vi "Track.vi"() -> ()   [LabVIEW 2014]
uses:
  <vilib>/Instr/_visa.llb/VISA Flush IO Buffer Mask.ctl
  <vilib>/Instr/_visa.llb/VISA Configure Serial Port (Instr).vi
panel:
  out "Direction":bool
  out "Whale?":bool
  out "read buffer":string
  out "return count":u32
  in  "stop":bool
  in  "VISA resource name":refnum<visa-resource-name>="COM3"
  in  "Base":dbl[][](array[numeric])
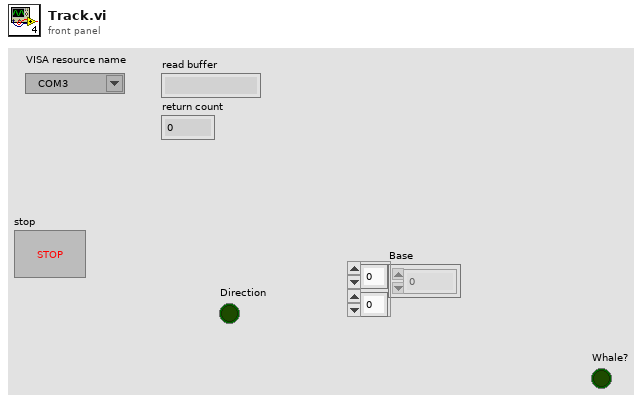
[diagram p1: front panel]
types:
  T1 = typedef "VISA Flush IO Buffer Mask.ctl" = u16
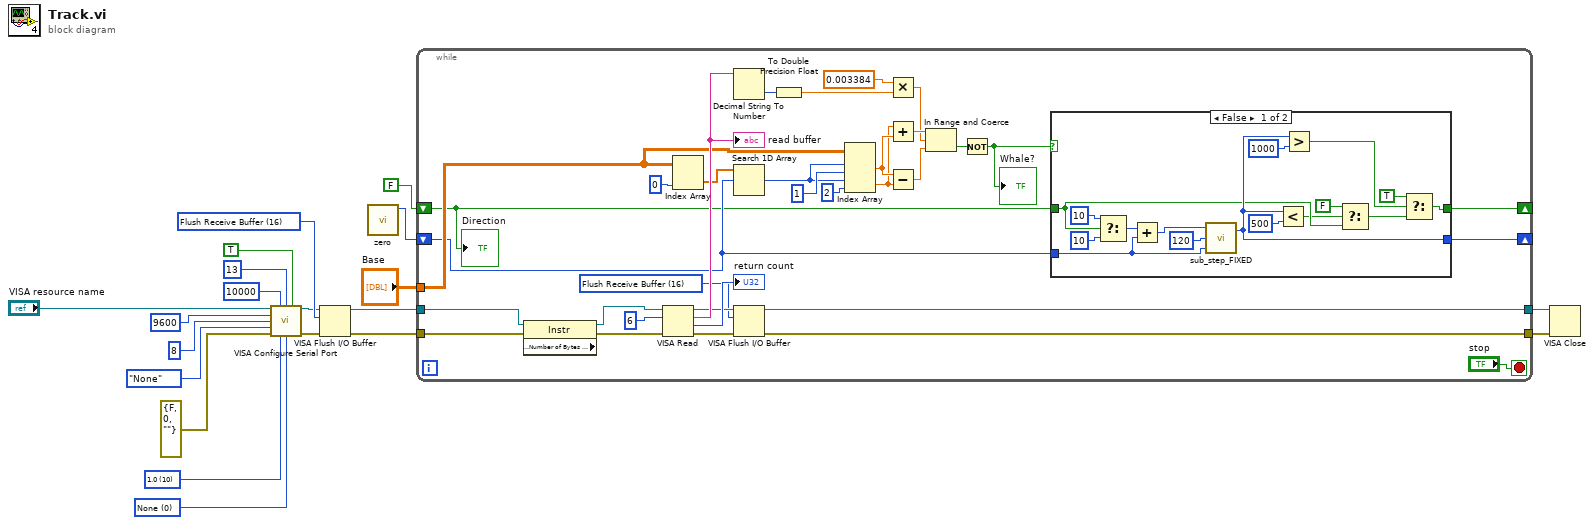
[diagram p0: block diagram]
diagram:
  w8 = T1 16 items=["Flush Receive Buffer"=16, "Write Transmit Buffer to Device"=32, "Flush Receive Buffer (No I/O)"=64, "Flush Transmit Buffer"=128] ("Mask")
  w14 = u16 0 items=["None", "XON/XOFF", "RTS/CTS", "XON/XOFF & RTS/CTS", "DTR/DSR", "XON/XOFF & DTR/DSR"] ("flow control (0:none)")
  w16 = u16 10 items=["1.0"=10, "1.5"=15, "2.0"=20] ("stop bits (10: 1 bit)")
  n1 = call-poly "VISA Configure Serial Port"("VISA resource name"="VISA resource name", "timeout (10sec)"=u32 10000, "termination char\n(0xA = '\\n' = LF)"=u8 13 ("termination char\n(0xA = '\\n' = LF)"), "Enable Termination\nChar (T)"=TRUE ("Enable Termination\nChar (T)"), "baud rate (9600)"=u32 9600, "data bits (8)"=u16 8, "parity (0:none)"=enum16{"None", "Odd", "Even", "Mark", "Space"}."None", "error in (no error)"=errorcluster {"status"=FALSE, "code"=0, "source"=""}, "stop bits (10: 1 bit)"=w16, "flow control (0:none)"=w14) -> ("VISA resource name out"=w7:refnum<visa-resource-name>, "error out"=w6:errorcluster)  [unwired: 4 in]
  n2 = VISA Flush I/O Buffer(VISA resource name=w7, mask (16)=w8, error in (no error)=w6) -> (VISA resource name out=w5:refnum<visa-resource-name>, error out=w4:errorcluster)
  n3 = call "zero.vi"() -> ("PositionOut"=w1:i32)  [unwired: 11 in]
  n4 = while {
    tunnel: [w44] -> w10
    tunnel: [w43] -> w9
    tunnel: w5 -> [w49]
    tunnel: w4 -> [w48]
    tunnel: "Base" -> [w34]
    shift-right: [w26] -> _
    shift-left: w1 -> [w27]
    shift-right: [w25] -> _
    shift-left: FALSE -> [w24]
    stop <- "stop" stop-if-true
    w40 = T1 16 items=["Flush Receive Buffer"=16, "Write Transmit Buffer to Device"=32, "Flush Receive Buffer (No I/O)"=64, "Flush Transmit Buffer"=128] ("Mask")
    n5 = property class="Instr" props=["Serial Settings:Number of Bytes at Serial Port"](reference=w49, error in=w48) -> (reference out=w53:refnum<visa-resource-name>, error out=w52:errorcluster)  [unwired: 1 out]
    n6 = VISA Read(VISA resource name=w53, byte count=u32 6, error in (no error)=w52) -> (VISA resource name out=w42:refnum<visa-resource-name>, read buffer=w50:string, return count=→"return count":u32, error out=w41:errorcluster)
    "read buffer" <- w50
    n7 = Index Array(array=w34, index (col)=u32 0 ("byte count")) -> (element=w36:dbl[])  [unwired: 1 in]
    n8 = Decimal String To Number(string=w50) -> (number=w47:i32)  [unwired: 2 in, 1 out]
    n9 = Search 1D Array(1D array=w36, element=w27) -> (index of element=w21:i32)  [unwired: 1 in]
    n10 = VISA Flush I/O Buffer(VISA resource name=w42, mask (16)=w40, error in (no error)=w41) -> (VISA resource name out=w44:refnum<visa-resource-name>, error out=w43:errorcluster)
    n11 = To Double Precision Float(number=w47) -> (double precision float=w46:dbl)
    n12 = Index Array(array=w34, index (row) #1=w21, index (col) #1=1 ("byte count"), index (row) #2=w21, index (col) #2=2 ("byte count")) -> (element #1=w33:dbl, element #2=w23:dbl)
    n13 = Multiply(x=0.003384, y=w46) -> (x*y=w30:dbl)
    n14 = Add(x=w23, y=w33) -> (x+y=w32:dbl)
    n15 = Subtract(x=w33, y=w23) -> (x-y=w31:dbl)
    n16 = In Range and Coerce(upper limit=w32, x=w30, lower limit=w31) -> (In Range?=w29:bool)  [unwired: 1 out]
    n17 = Not(x=w29) -> (.not. x?=w28:bool)
    "Whale?" <- w28
    n18 = case shown="False" w28 {
      tunnel: [w63 w71] -> w26
      tunnel: w27 -> [w68 w71]
      tunnel: [w58 w70] -> w25
      tunnel: w24 -> [w60 w70]
      frame False {
        n19 = Select(t=10 ("byte count"), s=w60, f=10 ("byte count")) -> (s? t:f=w69:i32)
        n20 = Add(x=w69, y=w68) -> (x+y=w67:i32)
        n21 = call "sub_step_FIXED.vi"("Current Position"=w68, "millisecond multiple"=u32 120 ("byte count"), "Desired Position"=w67) -> ("Position Out"=w63:i32)  [unwired: 1 in]
        n22 = Less?(x=w63, y=500 ("byte count")) -> (x < y?=w57:bool)
        n23 = Greater?(x=w63, y=1000 ("byte count")) -> (0:w56:bool)
        n24 = Select(t=FALSE, s=w57, f=w60) -> (s? t:f=w59:bool)
        n25 = Select(t=TRUE, s=w56, f=w59) -> (s? t:f=w58:bool)
      }
      frame True {
      }
    }
    "Direction" <- w24
  }
  n26 = VISA Close(VISA resource name=w10, error in (no error)=w9) -> ()  [unwired: 1 out]
